vi "test Add Find Remove Alias.vi"(8 "error in (no error)":errorcluster, 11 "TestCase in":refnum<class "Switch Scripting Unit Tests.lvclass">) -> (0 "error out":errorcluster, 3 "TestCase out":refnum<class "Switch Scripting Unit Tests.lvclass">)   [LabVIEW 2017, in "Switch Scripting Unit Tests.lvclass"]
uses:
  Switch Scripting Unit Tests.lvclass
  Shared/Alias Mapping.ctl
  Switch Scripting Unit Tests.lvclass/Switch Scripting Unit Tests.ctl
  <vilib>/addons/_JKI Toolkits/VI Tester/TestCase.llb/TestCase.lvclass
  Switch Scripting.lvlib
  Shared/Routing and Faulting Shared.lvlib
  C:/Program Files (x86)/National Instruments/LabVIEW 2017/vi.lib/addons/_JKI Toolkits/VI Tester/TestCase.llb/TestCase.lvclass
panel:
  in  "Save?":bool
  out "Output Filename":string
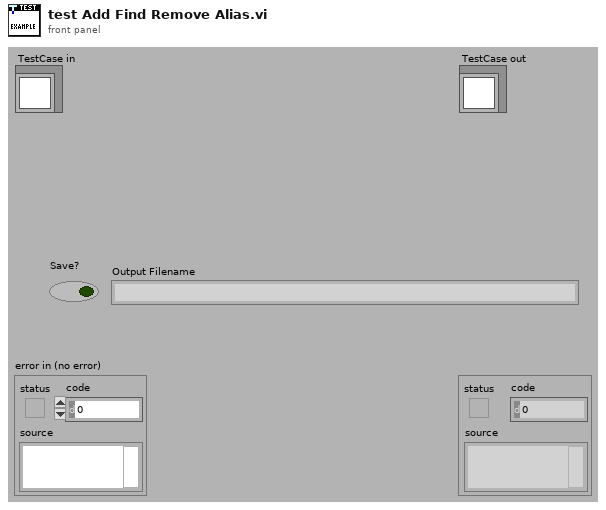
[diagram p1: front panel]
types:
  T1 = typedef "Routing and Faulting Shared.lvlib/Alias Mapping.ctl" = cluster{"Endpoint":string, "Alias":string}
  T2 = typedef "Custom Device API.lvlib/Custom Device Item Ref.ctl" = u64
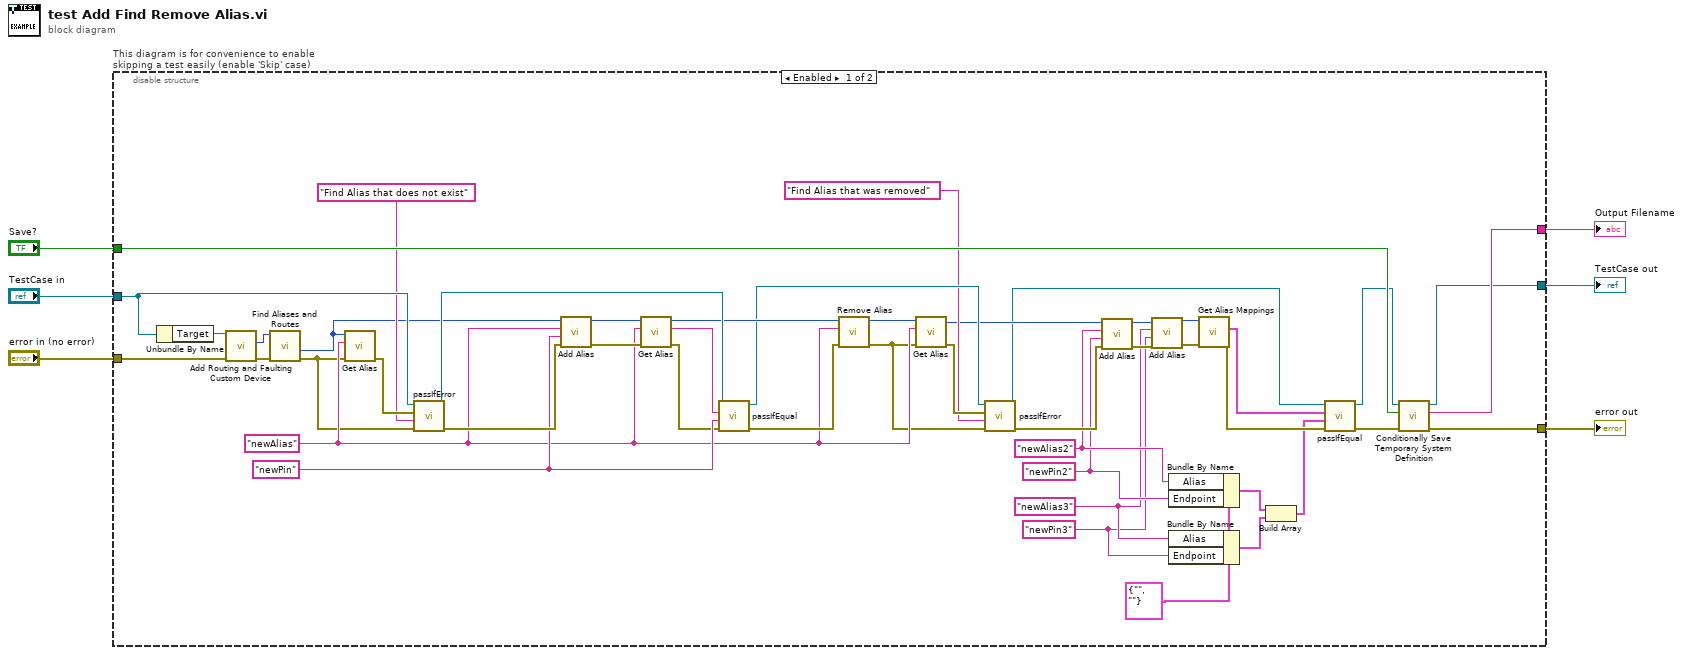
[diagram p0: block diagram]
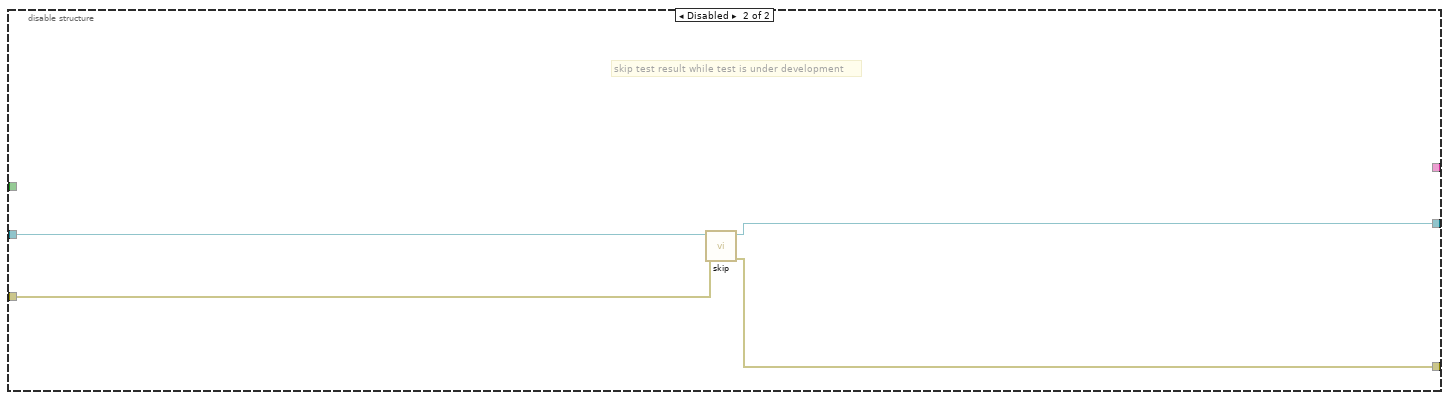
[diagram p2: hidden frame]
diagram:
  n1 = disable-structure "This diagram is for convenience to enable skipping a test easily (enable 'Skip' case)" shown="Enabled" {
    disable-tunnel: "TestCase in" -> [w47 w57]
    disable-tunnel: [w51 w55] -> w3
    disable-tunnel: [w52 w56] -> w5
    disable-tunnel: "error in (no error)" -> [w49 w54]
    disable-tunnel: [w53 _] -> w2
    disable-tunnel: "Save?" -> [w48 _]
    frame Enabled {
      w13 = T1 {"Endpoint"="", "Alias"=""} ("Alias Mapping")
      w14 = "newPin3" ("Alias")
      w15 = "newAlias3" ("Alias")
      w16 = "newPin2" ("Alias")
      w17 = "newAlias2" ("Alias")
      w39 = "newPin" ("Pin")
      w30 = "newAlias" ("Alias")
      n2 = Unbundle By Name(w47) -> ("Target"=w50:refnum<k24>)
      n3 = call "Add Routing and Faulting Custom Device.vi"("error in (no error)"=w49, "Target in"=w50) -> ("error out"=w44:errorcluster, "RaF CD Ref"=w8:T2)  [unwired: 7 in, 1 out]
      n4 = call "Find Aliases and Routes.vi"("error in (no error)"=w44, "RaF CD Ref in"=w8) -> ("error out"=w9:errorcluster, "Aliases Section Ref"=w7:T2)  [unwired: 6 in, 2 out]
      n5 = call "Get Alias.vi"("error in (no error)"=w9, "Alias"=w30, "Aliases Ref in"=w7) -> ("error out"=w46:errorcluster)  [unwired: 6 in, 2 out]
      n6 = call-dynamic "passIfError.vi"("error in (no error)"=w9, "task (\"\")"="Find Alias that does not exist" ("message (\"\")"), "error"=w46, "TestCase in"=w47) -> ("error out"=w43:errorcluster, "TestCase out"=w41:refnum<class "Switch Scripting Unit Tests.lvclass">)  [unwired: 6 in]
      n7 = call "Add Alias.vi"("error in (no error)"=w43, "Endpont"=w39, "Alias"=w30, "Aliases Ref in"=w7) -> ("error out"=w37:errorcluster, "Aliases Ref out"=w42:T2)  [unwired: 6 in]
      n8 = call "Get Alias.vi"("error in (no error)"=w37, "Alias"=w30, "Aliases Ref in"=w42) -> ("error out"=w38:errorcluster, "Endpont"=w40:string, "Aliases Ref out"=w36:T2)  [unwired: 6 in]
      n9 = call-dynamic "passIfEqual.vi"("error in (no error)"=w38, "y"=w39, "x"=w40, "TestCase in"=w41) -> ("error out"=w32:errorcluster, "TestCase out"=w34:refnum<class "Switch Scripting Unit Tests.lvclass">)  [unwired: 6 in]
      n10 = call "Remove Alias.vi"("error in (no error)"=w32, "Alias"=w30, "Aliases Ref in"=w36) -> ("error out"=w18:errorcluster, "Aliases Ref out"=w33:T2)  [unwired: 7 in]
      n11 = call "Get Alias.vi"("error in (no error)"=w18, "Alias"=w30, "Aliases Ref in"=w33) -> ("error out"=w35:errorcluster, "Aliases Ref out"=w29:T2)  [unwired: 6 in, 1 out]
      n12 = call-dynamic "passIfError.vi"("error in (no error)"=w18, "task (\"\")"="Find Alias that was removed" ("message (\"\")"), "error"=w35, "TestCase in"=w34) -> ("error out"=w28:errorcluster, "TestCase out"=w23:refnum<class "Switch Scripting Unit Tests.lvclass">)  [unwired: 6 in]
      n13 = call "Add Alias.vi"("error in (no error)"=w28, "Endpont"=w16, "Alias"=w17, "Aliases Ref in"=w29) -> ("error out"=w27:errorcluster, "Aliases Ref out"=w26:T2)  [unwired: 6 in]
      n14 = call "Add Alias.vi"("error in (no error)"=w27, "Endpont"=w14, "Alias"=w15, "Aliases Ref in"=w26) -> ("error out"=w24:errorcluster, "Aliases Ref out"=w25:T2)  [unwired: 6 in]
      n15 = Bundle By Name(cluster=w13, "Alias"=w17, "Endpoint"=w16) -> (w12:T1)
      n16 = Bundle By Name(cluster=w13, "Alias"=w15, "Endpoint"=w14) -> (w11:T1)
      n17 = call "Get Alias Mappings.vi"("error in (no error)"=w24, "Aliases Ref in"=w25) -> ("error out"=w20:errorcluster, "Alias Mappings"=w21:T1[])  [unwired: 7 in, 1 out]
      n18 = Build Array(w12, w11) -> (w10:T1[])
      n19 = call-dynamic "passIfEqual.vi"("error in (no error)"=w20, "y"=w10, "x"=w21, "TestCase in"=w23) -> ("error out"=w19:errorcluster, "TestCase out"=w22:refnum<class "Switch Scripting Unit Tests.lvclass">)  [unwired: 6 in]
      n20 = call "Conditionally Save Temporary System Definition.vi"("error in (no error)"=w19, "Save?"=w48, "Test Case"=w22) -> ("error out"=w52:errorcluster, "filename"=w53:string, "Test Case"=w51:refnum<class "Switch Scripting Unit Tests.lvclass">)  [unwired: 6 in]
    }
    frame Disabled {
      # "skip test result while test is under development"
      n21 = call <vilib>:"skip.vi"("error in (no error)"=w54, "TestCase in"=w57) -> ("error out"=w56:errorcluster, "TestCase out"=w55:refnum<class "Switch Scripting Unit Tests.lvclass">)  [unwired: 8 in]
    }
  }
  "error out" <- w5
  "TestCase out" <- w3
  "Output Filename" <- w2
